vi "svl_Exp Avg Resampled Level (1 Ch).vi"(5 "timeConstant":dbl=1.0 format="%.3f", 7 "exponential mode":enum16{"Slow", "Fast", "Impulse", "Custom"}(ring)=enum."Fast", 8 "error in (no error)":errorcluster, 9 "processing state":T1(ring), 11 "even angle signal":T2 {"even angle signal" format="%.2f"; "dr" format="%.2f"; "r0" format="%.2f"}) -> (0 "error out":errorcluster, 1 "dup processing state":T1(ring), 3 "even angle signal":T2 {"even angle signal" format="%.2f"; "dr" format="%.2f"; "r0" format="%.2f"}, 4 "actual time constant [ms]":dbl=125.0 format="%.2f")   [LabVIEW 2017]
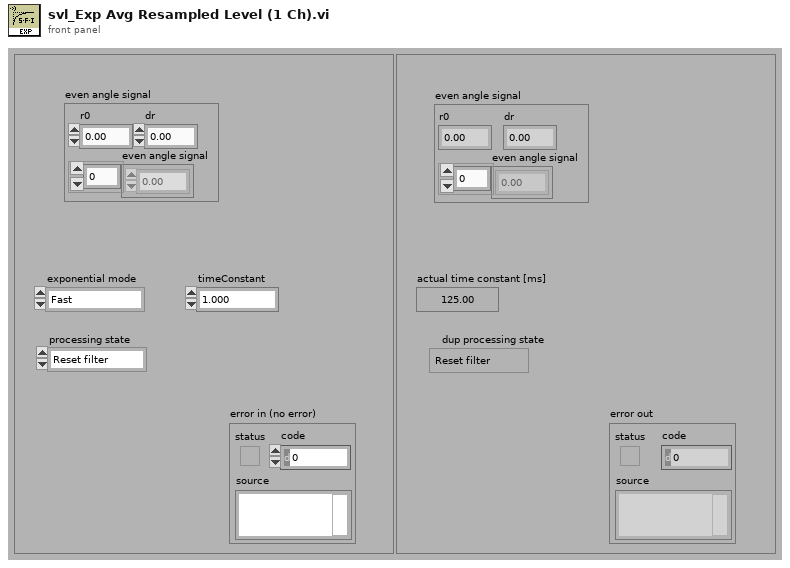
[diagram p1: front panel]
types:
  T1 = enum16{"Reset filter", "Restart averaging", "Continue processing"}
  T2 = cluster{"r0":dbl, "dr":dbl, "even angle signal":dbl[]}
  T3 = cluster{"Reverse Coefficients":dbl[], "Forward Coefficients":dbl[]}
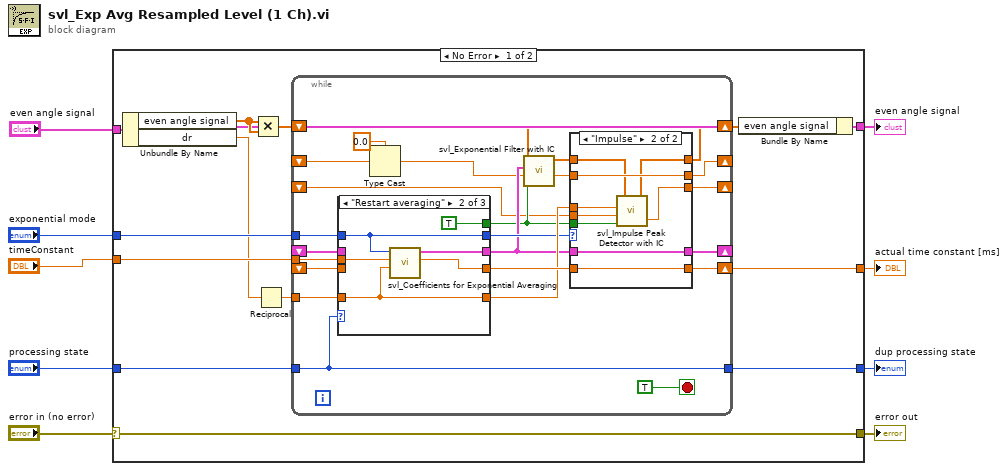
[diagram p0: block diagram]
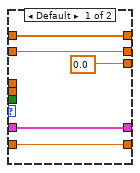
[diagram p2: hidden frame]
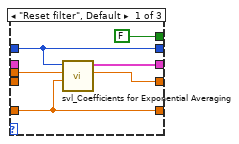
[diagram p3: hidden frame]
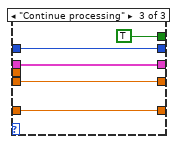
[diagram p4: hidden frame]
diagram:
  n1 = case shown="No Error" "error in (no error)" {
    selector: "error in (no error)" -> [w22 w81]
    tunnel: "even angle signal" -> [w10 w80]
    tunnel: "exponential mode" -> [w20 _]
    tunnel: "timeConstant" -> [w19 w79]
    tunnel: [w22 w81] -> w5
    tunnel: "processing state" -> [w21 w78]
    tunnel: [w12 w80] -> w3
    tunnel: [w17 w79] -> w2
    tunnel: [w16 w78] -> w1
    frame No Error {
      n2 = Unbundle By Name(w10) -> ("even angle signal"=w13:dbl[], "dr"=w14:dbl)
      n3 = Multiply(x=w13, y=w13) -> (x*y=w18:dbl[])
      n4 = Reciprocal(x=w14) -> (1/x=w15:dbl)
      n5 = while {
        tunnel: [w33] -> w16
        shift-left: _ -> [w43]
        shift-right: [w36] -> w17
        shift-left: _ -> [w44]
        shift-right: [w37] -> _
        shift-left: _ -> [w27]
        shift-right: [w38] -> _
        shift-left: _ -> [w24]
        shift-right: [w39] -> _
        tunnel: w15 -> [w26]
        tunnel: w19 -> [w46]
        tunnel: w20 -> [w42]
        tunnel: w21 -> [w33]
        shift-right: [w40] -> w11
        shift-left: w18 -> [w28]
        stop <- TRUE stop-if-true
        n6 = case shown="\"Restart averaging\"" w33 {
          tunnel: w42 -> [w62 w67 w73]
          tunnel: w46 -> [w66 w72 _]
          tunnel: w26 -> [w63 w69 w76]
          tunnel: [w65 w71 w75] -> w32
          tunnel: w44 -> [_ _ w75]
          tunnel: [w64 w68 w74] -> w41
          tunnel: w43 -> [_ _ w74]
          tunnel: [FALSE ("init/cont (init:F)") TRUE ("init/cont (init:F)") TRUE ("init/cont (init:F)")] -> w31
          tunnel: [w63 w69 w76] -> w35
          tunnel: [w62 w67 w73] -> w34
          frame "Reset filter", Default {
            n7 = call <vilib>:"svl_Coefficients for Exponential Averaging.vi"("sampling frequency [Hz]"=w63, "time constant [ms]"=w66, "exponential mode"=w62) -> ("actual time constant [ms]"=w64:dbl, "filter coefficients"=w65:T3)  [unwired: 3 in]
          }
          frame "Restart averaging" {
            n8 = call <vilib>:"svl_Coefficients for Exponential Averaging.vi"("sampling frequency [Hz]"=w69, "time constant [ms]"=w72, "exponential mode"=w67) -> ("actual time constant [ms]"=w68:dbl, "filter coefficients"=w71:T3)  [unwired: 3 in]
          }
          frame "Continue processing" {
          }
        }
        n9 = Type Cast(type=0.0 ("final filter state"), x=w24) -> (*(type *) &x=w23:dbl)
        n10 = call <vilib>:"svl_Exponential Filter with IC.vi"("init/cont (init:F)"=w31, "initial filter state"=w23, "filter coefficients"=w32, "X"=w28) -> ("final filter state"=w29:dbl, "filtered X"=w30:dbl[])  [unwired: 5 in, 1 out]
        n11 = case shown="\"Impulse\"" w34 {
          tunnel: w30 -> [w50 w59]
          tunnel: w29 -> [w51 w60]
          tunnel: [w51 w60] -> w39
          tunnel: w35 -> [_ w58]
          tunnel: w31 -> [_ w57]
          tunnel: [0.0 ("final filter state") w56] -> w38
          tunnel: [w50 w55] -> w40
          tunnel: w41 -> [w49 w54]
          tunnel: [w49 w54] -> w36
          tunnel: w32 -> [w48 w53]
          tunnel: [w48 w53] -> w37
          tunnel: w27 -> [_ w52]
          frame Default {
          }
          frame "Impulse" {
            n12 = call <vilib>:"svl_Impulse Peak Detector with IC.vi"("init/cont (init:F)"=w57, "initial filter state"=w52, "sampling frequency [Hz]"=w58, "X"=w59) -> ("final filter state"=w56:dbl, "filtered X"=w55:dbl[])
          }
        }
      }
      n13 = Bundle By Name(cluster=w10, "even angle signal"=w11) -> (w12:T2)
    }
    frame Error {
    }
  }
  "even angle signal" <- w3
  "error out" <- w5
  "actual time constant [ms]" <- w2
  "dup processing state" <- w1
